vi "Circle_flicker_for_perimetry.vi"(8 "shiftY":dbl, 9 "shiftX":dbl, 11 "Min&Max Voltage":dbl=0.025) -> (0 "Rate":dbl=12800.0, 2 "Scanners trajectories":dbl[][](graph), 3 "XY Graph":cluster{"sine wave":dbl[], "sine wave":dbl[]}(graph)={"sine wave"=[0.0, 0.0012266918581854505, 0.0024504285082390153, 0.003668261861384044, 0.0048772580504032065, 0.006074504497581597, 0.007257116931361559, 0.0084222463348055, 0.009567085809127244, 0.010688877335757052, 0.01178491842064994, 0.012852568604830542, 0.013889255825490054, 0.014892482612310833, 0.015859832104091136, 0.01678897387117546, 0.017677669529663688, 0.01852377813387398, 0.019325261334068422, 0.020080188287016125, 0.02078674030756363, 0.021443215250006805, 0.022048031608708874, 0.022599732328086087, 0.023096988312782167, 0.023538601629575523, 0.023923508393305218, 0.024250781329863604, 0.02451963201008076, 0.02472941274911953, 0.02487961816680492, 0.024969886405129316, 0.024999999999999998, 0.024969886405129316, 0.02487961816680492, 0.02472941274911953, 0.02451963201008076, 0.024250781329863604, 0.023923508393305218, 0.023538601629575523, 0.023096988312782164, 0.022599732328086087, 0.02204803160870887, 0.021443215250006805, 0.020786740307563625, 0.020080188287016125, 0.01932526133406842, 0.01852377813387398, 0.017677669529663684, 0.01678897387117546, 0.015859832104091136, 0.014892482612310833, 0.013889255825490054, 0.012852568604830542, 0.01178491842064994, 0.01068887733575705, 0.009567085809127244, 0.008422246334805499, 0.007257116931361559, 0.0060745044975815945, 0.0048772580504032065, 0.0036682618613840404, 0.002450428508239015, 0.0012266918581854466, 0.0, -0.0012266918581854548, -0.002450428508239015, -0.0036682618613840486, -0.0048772580504032065, -0.006074504497581602, -0.007257116931361558, -0.008422246334805508, -0.009567085809127244, -0.010688877335757059, -0.01178491842064994, -0.01285256860483055, -0.013889255825490054, -0.014892482612310841, -0.015859832104091136, -0.016788973871175467, -0.017677669529663684, -0.018523778133873986, -0.01932526133406842, -0.020080188287016132, -0.020786740307563625, -0.021443215250006812, -0.02204803160870887, -0.022599732328086094, -0.023096988312782164, -0.02353860162957553, -0.023923508393305218, -0.02425078132986361, -0.02451963201008076, -0.024729412749119536, -0.02487961816680492, -0.024969886405129323, -0.024999999999999998, -0.024969886405129323, -0.02487961816680492, -0.024729412749119536, -0.02451963201008076, -0.02425078132986361, -0.023923508393305218, -0.02353860162957553, -0.023096988312782164, -0.022599732328086094, -0.02204803160870887, -0.021443215250006812, -0.020786740307563625, -0.020080188287016132, -0.01932526133406842, -0.018523778133873986, -0.017677669529663684, -0.016788973871175467, -0.015859832104091136, -0.01489248261231084, -0.013889255825490054, -0.012852568604830547, -0.01178491842064994, -0.010688877335757054, -0.009567085809127244, -0.0084222463348055, -0.007257116931361559, -0.0060745044975815945, -0.0048772580504032065, -0.003668261861384039, -0.002450428508239015, -0.0012266918581854435], "sine wave"=[0.025, 0.024969886405129312, 0.024879618166804923, 0.024729412749119526, 0.024519632010080762, 0.0242507813298636, 0.02392350839330522, 0.02353860162957552, 0.023096988312782167, 0.022599732328086083, 0.022048031608708874, 0.0214432152500068, 0.02078674030756363, 0.02008018828701612, 0.019325261334068422, 0.018523778133873976, 0.017677669529663688, 0.016788973871175457, 0.015859832104091136, 0.01489248261231083, 0.013889255825490054, 0.012852568604830542, 0.01178491842064994, 0.01068887733575705, 0.009567085809127244, 0.008422246334805499, 0.007257116931361558, 0.006074504497581595, 0.004877258050403205, 0.003668261861384042, 0.0024504285082390127, 0.0012266918581854487, -3.0357660829594124e-18, -0.0012266918581854518, -0.0024504285082390187, -0.003668261861384045, -0.004877258050403211, -0.006074504497581599, -0.0072571169313615635, -0.008422246334805502, -0.009567085809127249, -0.010688877335757054, -0.011784918420649947, -0.012852568604830543, -0.013889255825490061, -0.014892482612310833, -0.015859832104091143, -0.016788973871175457, -0.017677669529663695, -0.018523778133873972, -0.01932526133406843, -0.020080188287016118, -0.020786740307563636, -0.021443215250006798, -0.02204803160870888, -0.02259973232808608, -0.023096988312782174, -0.023538601629575516, -0.023923508393305225, -0.024250781329863597, -0.024519632010080766, -0.024729412749119523, -0.024879618166804927, -0.02496988640512931, -0.025, -0.02496988640512931, -0.024879618166804923, -0.024729412749119523, -0.024519632010080762, -0.024250781329863597, -0.02392350839330522, -0.023538601629575516, -0.023096988312782167, -0.02259973232808608, -0.022048031608708874, -0.021443215250006798, -0.02078674030756363, -0.020080188287016118, -0.019325261334068422, -0.018523778133873972, -0.017677669529663684, -0.016788973871175457, -0.015859832104091132, -0.01489248261231083, -0.01388925582549005, -0.012852568604830542, -0.011784918420649933, -0.010688877335757052, -0.009567085809127235, -0.0084222463348055, -0.00725711693136155, -0.006074504497581597, -0.004877258050403196, -0.003668261861384044, -0.0024504285082390044, -0.0012266918581854505, 1.0842021724855044e-17, 0.00122669185818545, 0.002450428508239026, 0.0036682618613840434, 0.004877258050403218, 0.006074504497581597, 0.00725711693136157, 0.0084222463348055, 0.009567085809127256, 0.010688877335757052, 0.011784918420649953, 0.012852568604830542, 0.013889255825490067, 0.01489248261231083, 0.01585983210409115, 0.016788973871175457, 0.017677669529663702, 0.018523778133873972, 0.019325261334068436, 0.020080188287016118, 0.020786740307563643, 0.021443215250006798, 0.022048031608708888, 0.02259973232808608, 0.02309698831278218, 0.023538601629575516, 0.02392350839330523, 0.024250781329863597, 0.02451963201008077, 0.024729412749119523, 0.02487961816680493, 0.02496988640512931]})   [LabVIEW 2021]
uses:
  <vilib>/Analysis/1siggen.llb/Ramp Pattern by Samples.vi
  <vilib>/Analysis/NI_AALBase.lvlib
panel:
  out "Cycle duration":i32=128
  out "output array":dbl[][](array[numeric])
  in  "Number of cycles":i32=20
  # "Ta wersja Flicker circle zakłada,  ze skanery są cały czas w tle (x = 0V, Y = -4V), wyprowadza je z tła i kończy w tle."
  # "Przy 12800 S/s i 128 sampli na bodziec, czas trwania 1 cyklu 10 ms"
  # "przerwa w tle ustawiona na 600 ms"
  # "Dodatkowo najazdy trwają 2 razy po 1,5 ms"
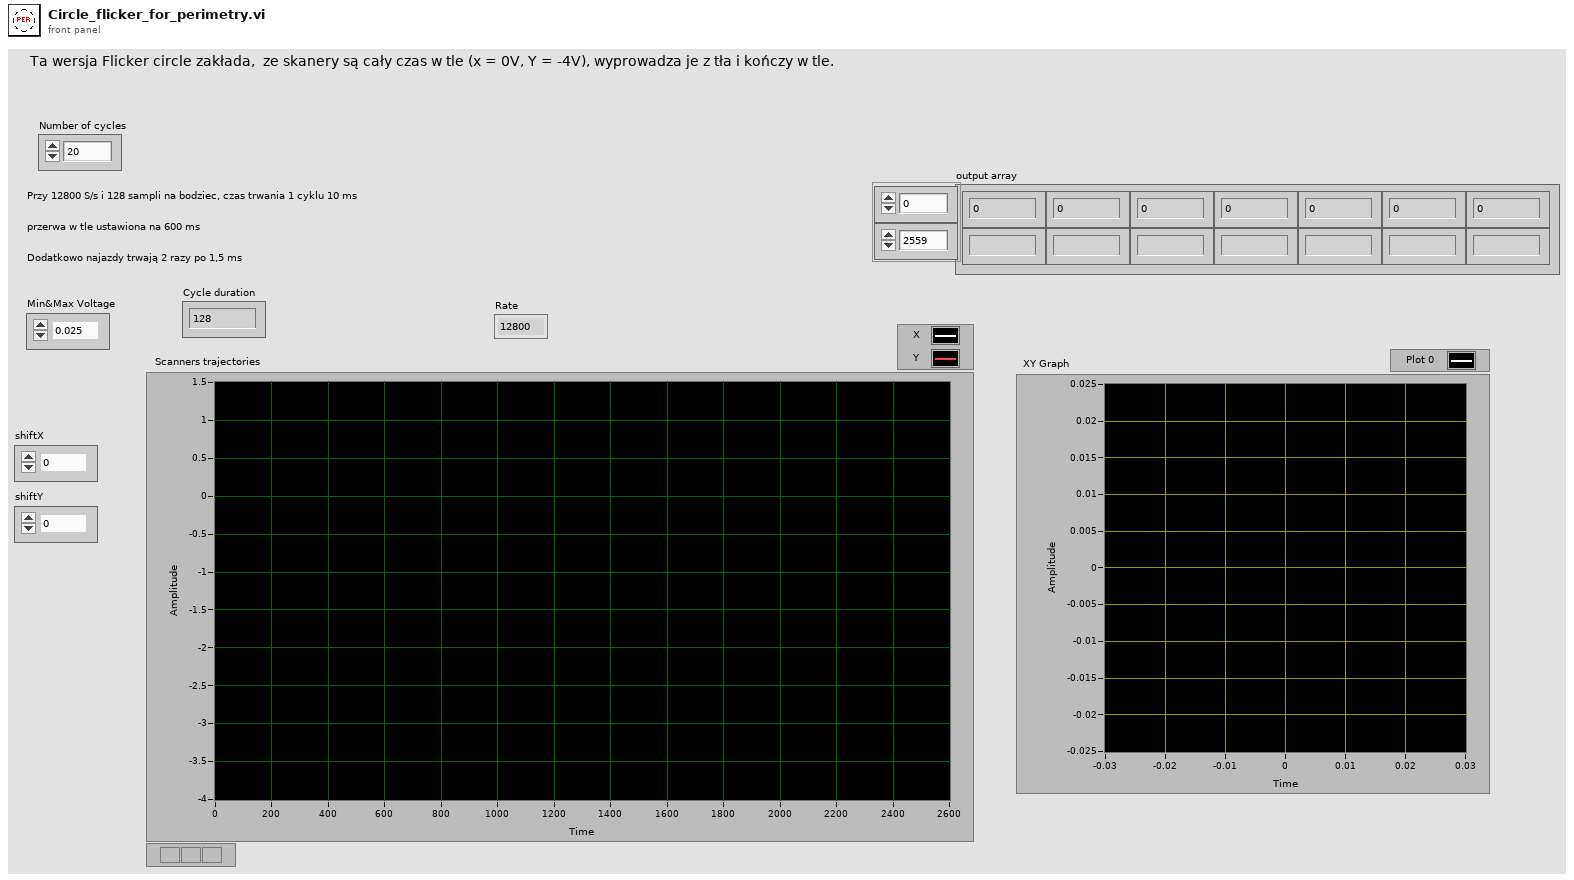
[diagram p1: front panel]
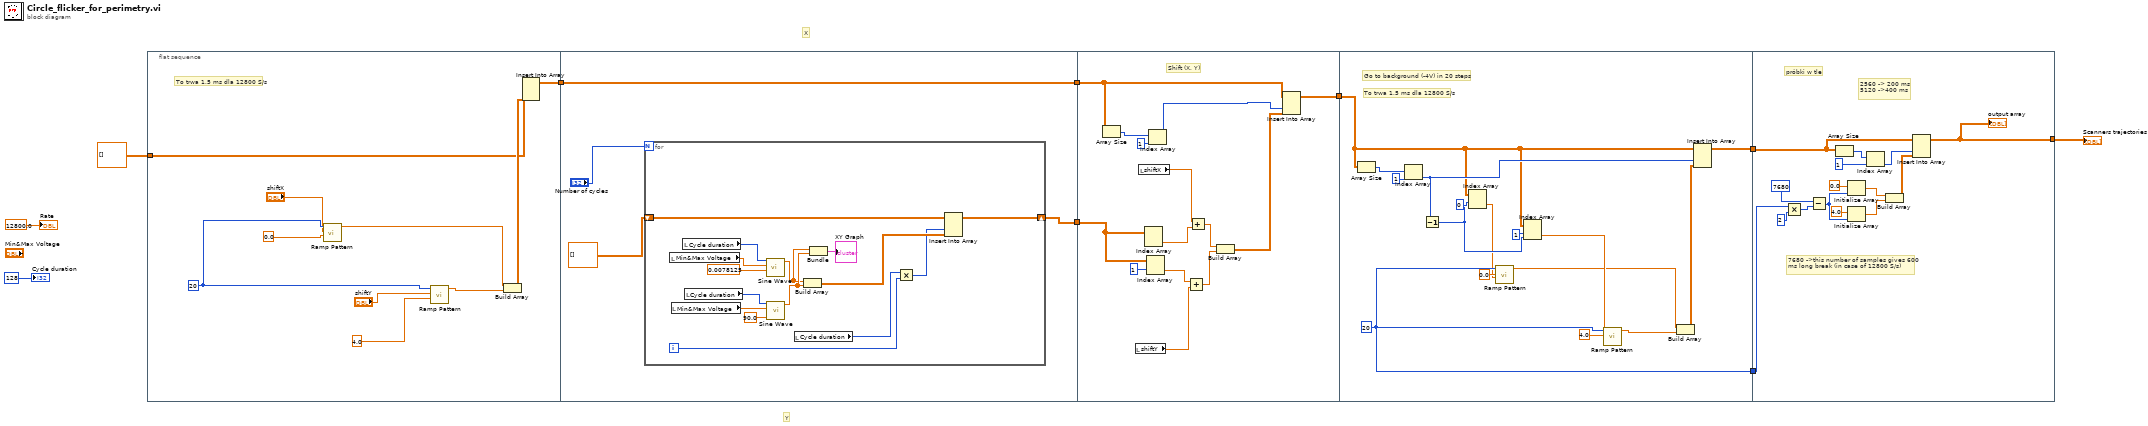
[diagram p0: block diagram]
diagram:
  # "Y"
  # "X"
  n1 = flat-sequence {
    tunnel: dbl[][] [] -> [w16]
    tunnel: [w11] -> w3
    tunnel: [w22] -> w6
    tunnel: w3 -> [w21]
    tunnel: [w21] -> w2
    tunnel: w6 -> [w48]
    tunnel: [w45] -> w5
    tunnel: w2 -> [w41]
    tunnel: w5 -> [w57]
    tunnel: [w64] -> w10
    tunnel: [w60] -> w7
    tunnel: w7 -> [w79]
    tunnel: w10 -> [w73]
    tunnel: [w70] -> w1
    frame #0 {
      w18 = 20 ("dimension size")
      # "To trwa 1,5 ms dla 12800 S/s"
      n2 = call-poly <vilib>:"Ramp Pattern.vi"("start"=0.0 ("element"), "end"="shiftX", "samples"=w18) -> ("Ramp Pattern"=w17:dbl[])  [unwired: 7 in, 1 out]
      n3 = call-poly <vilib>:"Ramp Pattern.vi"("start"=4.0 ("end"), "end"="shiftY", "samples"=w18) -> ("Ramp Pattern"=w20:dbl[])  [unwired: 7 in, 1 out]
      n4 = Build Array(w17, w20) -> (w19:dbl[][])
      n5 = Insert Into Array(array=w16, new element=w19) -> (w11:dbl[][])  [unwired: 2 in]
    }
    frame #1 {
      n6 = for {
        N: "Number of cycles" -> [_]
        shift-right: [w35] -> w22
        shift-left: dbl[][] [] -> [w37]
        i -> [w33]
        n7 = local read "Min&Max Voltage"() -> (w32:dbl)
        n8 = local read "Min&Max Voltage"() -> (w31:dbl)
        n9 = local read "Cycle duration"() -> (w30:i32)
        n10 = local read "Cycle duration"() -> (w29:i32)
        n11 = call <vilib>:"Sine Wave.vi"("samples"=w30, "amplitude"=w32, "frequency"=0.0078125) -> ("sine wave"=w26:dbl[])  [unwired: 2 in, 2 out]
        n12 = call <vilib>:"Sine Wave.vi"("samples"=w29, "amplitude"=w31, "phase in"=90.0) -> ("sine wave"=w27:dbl[])  [unwired: 2 in, 2 out]
        n13 = local read "Cycle duration"() -> (w28:i32)
        n14 = Build Array(w26, w27) -> (w36:dbl[][])
        n15 = Bundle("sine wave"=w26, "sine wave"=w27) -> (→"XY Graph":cluster{"sine wave":dbl[], "sine wave":dbl[]})  [unwired: 1 in]
        n16 = Multiply(x=w28, y=w33) -> (x*y=w34:i32)
        n17 = Insert Into Array(array=w37, index (col)=w34, new element=w36) -> (w35:dbl[][])  [unwired: 1 in]
      }
    }
    frame #2 {
      # "Shift (X, Y)"
      n18 = Array Size(array=w41) -> (size(s)=w43:i32[])
      n19 = local read "shiftY"() -> (w46:dbl)
      n20 = local read "shiftX"() -> (w47:dbl)
      n21 = Index Array(array=w48) -> (element=w50:dbl[])  [unwired: 2 in]
      n22 = Index Array(array=w48, index (row)=1) -> (element=w51:dbl[])  [unwired: 1 in]
      n23 = Index Array(array=w43, index=1) -> (element=w40:i32)
      n24 = Add(x=w51, y=w46) -> (x+y=w53:dbl[])
      n25 = Add(x=w47, y=w50) -> (x+y=w52:dbl[])
      n26 = Build Array(w52, w53) -> (w44:dbl[][])
      n27 = Insert Into Array(array=w41, index (col)=w40, new element=w44) -> (w45:dbl[][])  [unwired: 1 in]
    }
    frame #3 {
      w60 = 20 ("dimension size")
      # "To trwa 1,5 ms dla 12800 S/s"
      # "Go to background (-4V) in 20 steps"
      n28 = Array Size(array=w57) -> (size(s)=w67:i32[])
      n29 = Index Array(array=w67, index=1) -> (element=w63:i32)
      n30 = Decrement(x=w63) -> (x-1=w56:i32)
      n31 = Index Array(array=w57, index (row)=0, index (col)=w56) -> (element=w55:dbl)
      n32 = call-poly <vilib>:"Ramp Pattern.vi"("start"=w55, "end"=0.0 ("element"), "samples"=w60) -> ("Ramp Pattern"=w54:dbl[])  [unwired: 7 in, 1 out]
      n33 = Index Array(array=w57, index (row)=1 ("disabled index (row)"), index (col)=w56) -> (element=w61:dbl)
      n34 = call-poly <vilib>:"Ramp Pattern.vi"("start"=w61, "end"=4.0, "samples"=w60) -> ("Ramp Pattern"=w68:dbl[])  [unwired: 7 in, 1 out]
      n35 = Build Array(w54, w68) -> (w65:dbl[][])
      n36 = Insert Into Array(array=w57, index (col)=w63, new element=w65) -> (w64:dbl[][])  [unwired: 1 in]
    }
    frame #4 {
      # "2560 -> 200 ms\n5120 ->400 ms"
      # "7680 ->this number of samples gives 600 ms long break (in case of 12800 S/s)"
      # "próbki w tle"
      n37 = Multiply(x=w79, y=2) -> (x*y=w77:i32)
      n38 = Subtract(x=7680 ("Numeric Control"), y=w77) -> (x-y=w76:i32)
      n39 = Array Size(array=w73) -> (size(s)=w75:i32[])
      n40 = Initialize Array(0.0 ("element"), w76) -> (w82:dbl[])
      n41 = Initialize Array(4.0 ("element"), w76) -> (w81:dbl[])
      n42 = Index Array(array=w75, index=1) -> (element=w72:i32)
      n43 = Build Array(w82, w81) -> (w71:dbl[][])
      n44 = Insert Into Array(array=w73, index (col)=w72, new element=w71) -> (w70:dbl[][])  [unwired: 1 in]
      "output array" <- w70
    }
  }
  "Scanners trajectories" <- w1
  "Rate" <- 12800.0 ("Rate")
  "Cycle duration" <- 128
